vi "DropDetectionForLinkam ver 3.vi"(0 "Range (Threshold 1)":cluster{"Lower value":sgl, "Upper value":sgl}={"Lower value"=76.0, "Upper value"=255.0}, 1 "Min Radius (Circle Detection 1)":sgl=3.0, 2 "Max Radius (Circle Detection 1)":sgl=500.0, 7 "error in":errorcluster) -> (20 "Nb Circles (Circle Detection 1)":i32, 21 "Circles Data (Circle Detection 1)":T2(array[cluster]), 22 "Circles Data (calibrated) (Circle Detection 1)":T2(array[cluster]), 27 "error out":errorcluster)   [LabVIEW 2013]
uses:
  <vilib>/vision/NI_Vision_Development_Module.lvlib
panel:
  out "Image Out":T1(plugin-control)
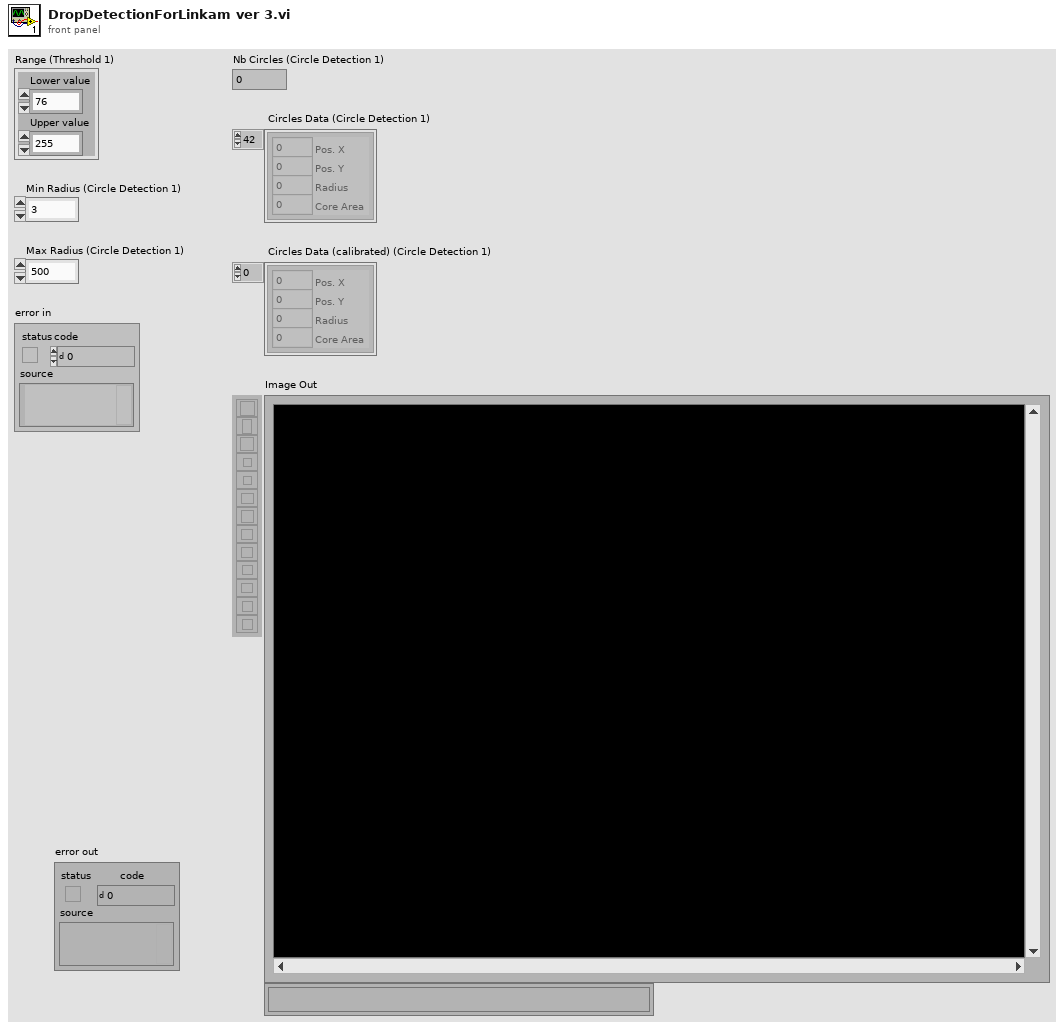
[diagram p1: front panel]
types:
  T1 = typedef "IMAQ Image.ctl" = refnum<image>
  T2 = cluster{"Pos. X":i32, "Pos. Y":i32, "Radius":i32, "Core Area":i32}[]
  T3 = cluster{"Global Rectangle":i32[], "Contours":cluster{"ID":enum32{"External", "Internal"}, "Type":u32, "Coordinates":i32[]}[]}
  T4 = typedef "Image Type" = u32
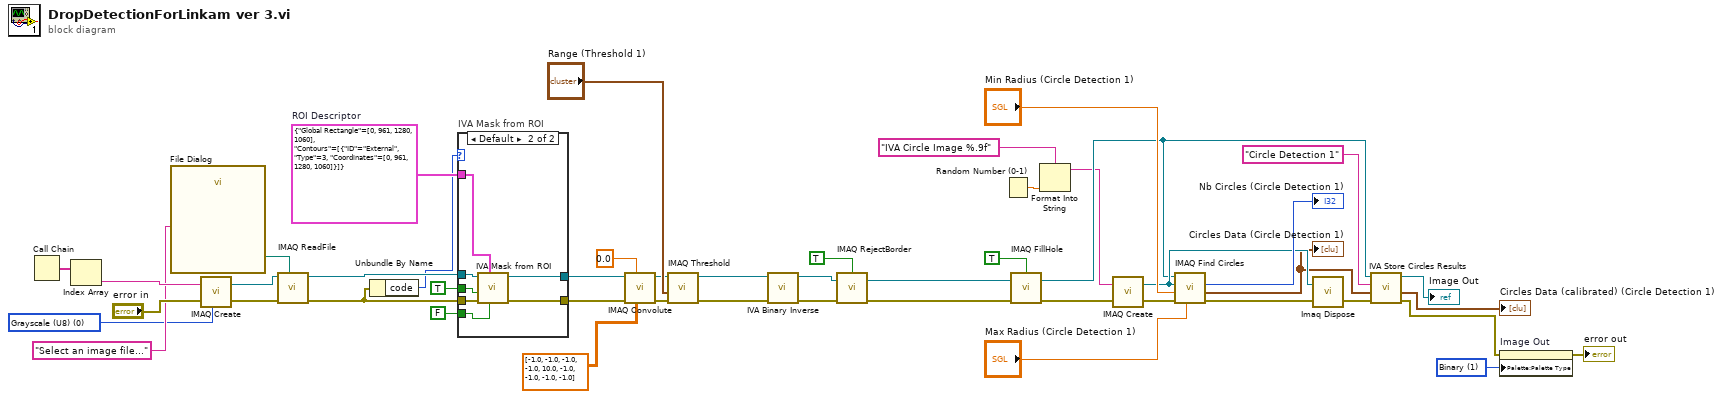
[diagram p0: block diagram]
diagram:
  w3 = u32 1 items=["Grayscale", "Binary", "Gradient", "Rainbow", "Temperature", "User Defined"] ("Palette")
  w40 = T3 {"Global Rectangle"=[0, 961, 1280, 1060], "Contours"=[{"ID"=enum."External", "Type"=3, "Coordinates"=[0, 961, 1280, 1060]}]}  # ROI Descriptor
  w41 = T4 0 items=["Grayscale (U8)", "Grayscale (I16)", "Grayscale (SGL)", "Complex (CSG)", "RGB (U32)", "HSL (U32)", "RGB (U64)", "Grayscale (U16)"] ("Image Type")
  n1 = Call Chain() -> (call chain=w45:string[])
  n2 = Index Array(array=w45) -> (element=w44:string)  [unwired: 1 in]
  n3 = call "File Dialog"("prompt"="Select an image file...") -> ("selected path"=w42:path)  [unwired: 6 in, 8 out]
  n4 = call "IMAQ Create"("Image Name"=w44, "Image Type"=w41, "error in (no error)"="error in") -> ("New Image"=w48:T1, "error out"=w47:errorcluster)  [unwired: 1 in, 1 out]
  n5 = call "IMAQ ReadFile"("File Path"=w42, "error in (no error)"=w47, "Image"=w48) -> ("error out"=w36:errorcluster, "Image Out"=w38:T1)  [unwired: 2 in, 5 out]
  n6 = Unbundle By Name(w36) -> ("code"=w35:i32)
  n7 = case "IVA Mask from ROI" shown="Default" w35 {
    tunnel: w40 -> [_ w56]
    tunnel: FALSE ("Shrink") -> [_ w55]
    tunnel: w38 -> [w49 w54]
    tunnel: w36 -> [_ w53]
    tunnel: [_ w52] -> w32
    tunnel: [w49 w51] -> w33
    tunnel: TRUE ("Out / In") -> [_ w50]
    frame -1074396199, -1074396198 {
      # "Discard\nCoordinate\nSystem\nError"
    }
    frame Default {
      n8 = call <vilib>:"IVA Mask from ROI.vi"("Shrink"=w55, "ROI Descriptor"=w56, "error in (no error)"=w53, "Out / In"=w50, "Image Src"=w54) -> ("error out"=w52:errorcluster, "Image Out"=w51:T1)  [unwired: 5 out]
    }
  }
  n9 = call "IMAQ Convolute"("Kernel"=sgl[][] [[-1.0, -1.0, -1.0], [-1.0, 10.0, -1.0], [-1.0, -1.0, -1.0]], "Divider (kernel sum)"=sgl 0.0 ("Divider"), "error in (no error)"=w32, "Image Src"=w33) -> ("error out"=w28:errorcluster, "Image Dst Out"=w29:T1)  [unwired: 3 in, 3 out]
  n10 = call "IMAQ Threshold"("error in (no error)"=w28, "Range"="Range (Threshold 1)", "Image Src"=w29) -> ("error out"=w26:errorcluster, "Image Dst Out"=w27:T1)  [unwired: 3 in, 4 out]
  n11 = call <vilib>:"IVA Binary Inverse.vi"("error in (no error)"=w26, "Image In"=w27) -> ("error out"=w23:errorcluster, "Image Out"=w24:T1)  [unwired: 8 out]
  n12 = call "IMAQ RejectBorder"("error in (no error)"=w23, "Image Src"=w24, "Connectivity 4/8 (8)"=TRUE) -> ("error out"=w20:errorcluster, "Image Dst Out"=w21:T1)  [unwired: 1 in, 2 out]
  n13 = Random Number (0-1)() -> (number: 0 to 1=w5:dbl)
  n14 = call "IMAQ FillHole"("error in (no error)"=w20, "Image Src"=w21, "Connectivity 4/8 (8)"=TRUE) -> ("error out"=w14:errorcluster, "Image Dst Out"=w11:T1)  [unwired: 1 in, 2 out]
  n15 = Format Into String(format string="IVA Circle Image %.9f" ("Image Name"), w5) -> (resulting string=w7:string)  [unwired: 2 in, 1 out]
  n16 = call "IMAQ Create"("Image Name"=w7, "error in (no error)"=w14) -> ("New Image"=w16:T1, "error out"=w15:errorcluster)  [unwired: 2 in, 1 out]
  n17 = call "IMAQ Find Circles"("Max Radius"="Max Radius (Circle Detection 1)", "error in (no error)"=w15, "Min Radius"="Min Radius (Circle Detection 1)", "Image Dst"=w16, "Image Src"=w11) -> ("error out"=w13:errorcluster, "Circles Data"=w9:T2, "Nb Circles"=→"Nb Circles (Circle Detection 1)":i32)  [unwired: 4 out]
  "Circles Data (Circle Detection 1)" <- w9
  n18 = call "Imaq Dispose"("Image"=w16, "error in (no error)"=w13) -> ("error out"=w12:errorcluster)  [unwired: 1 in, 3 out]
  n19 = call <vilib>:"IVA Store Circles Results.vi"("error in (no error)"=w12, "Circles Data"=w9, "Step Name"="Circle Detection 1", "Image in"=w11) -> ("error out"=w2:errorcluster, "Circles Data (calibrated)"=→"Circles Data (calibrated) (Circle Detection 1)":T2, "Image dup"=→"Image Out":T1)  [unwired: 5 out]
  n20 = property on="Image Out" class="ImageControl"(error in=w2, "Palette:Palette Type"=w3) -> (error out=→"error out":errorcluster)  [unwired: 1 in, 1 out]
